vi "error_window.vi"(7 "callee":refnum<vi>, 8 "error in (no error)":errorcluster, 11 "v1 in":refnum<class "v1.lvclass">) -> (0 "error out":errorcluster, 2 "dialog_selection":T1=enum."button_2", 3 "v1 out":refnum<class "v1.lvclass">)   [LabVIEW 2015, in "lv-dialog-interfaces.lvlib" / "v1.lvclass"]
uses:
  v1.lvclass
  lv-dialog/api/v1/public/_controls/dialog_selection.ctl
  <vilib>/Utility/error.llb/DialogTypeEnum.ctl
  lv-dialog-interfaces.lvlib
  lv-dialog/api/v1/v1.lvlib
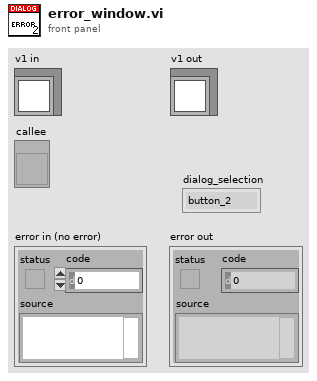
[diagram p1: front panel]
types:
  T1 = typedef "lv-dialog.lvlib/v1.lvlib/dialog_selection.ctl" = enum16{"null", "panel_closed", "button_1", "button_2", "button_3", "cancelled"}
  T2 = typedef "DialogTypeEnum.ctl" = enum16{"no dialog", "OK message", "continue or stop message", "auto error handling dialog", "OK message + warnings", "continue/stop + warnings"}
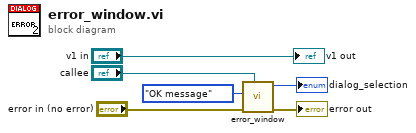
[diagram p0: block diagram]
diagram:
  n1 = call "error_window.vi"("calling_vi"="callee", "error in (no error)"="error in (no error)", "dialog type"=DialogTypeEnum."OK message") -> ("error out"=→"error out":errorcluster, "dialog_selection"=→"dialog_selection":T1)  [unwired: 7 in]
  "v1 out" <- "v1 in"
